vi "Table_BCK_Push.vi"(8 "error in (no error)":errorcluster, 11 "index":i32) -> (0 "Tables[]":string[](array[string]), 3 "Table Name":string)   [LabVIEW 2020]
uses:
  MS SQL/MS_Global.vi
panel:
  out "error out":errorcluster
  # "BCK_OP80_08_ASR"
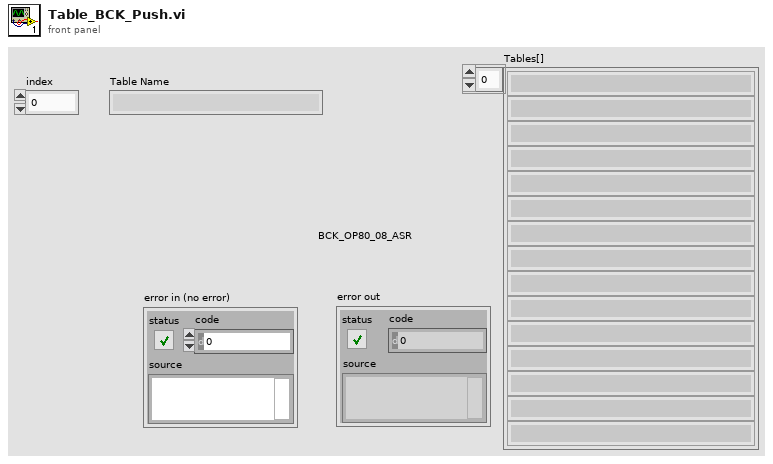
[diagram p1: front panel]
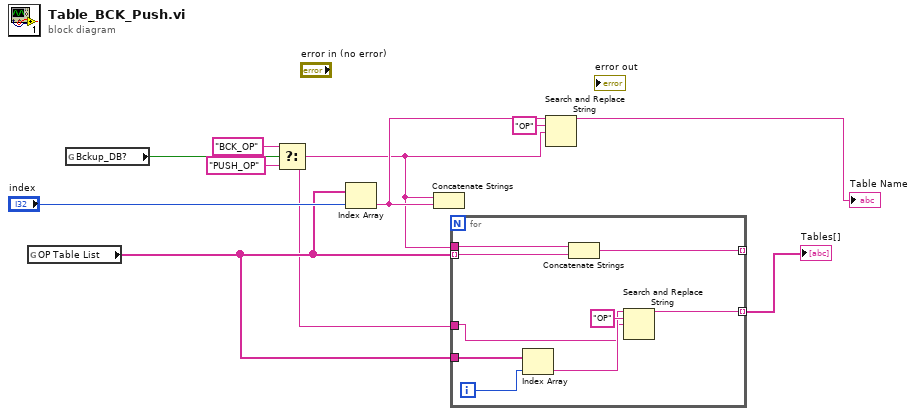
[diagram p0: block diagram]
diagram:
  n1 = global read "MS_Global.vi" "OP Table List"() -> (w5:string[])
  n2 = global read "MS_Global.vi" "Bckup_DB?"() -> (w7:bool)
  n3 = Select(t="BCK_OP", s=w7, f="PUSH_OP") -> (s? t:f=w2:string)
  n4 = Index Array(array=w5, index="index") -> (element=w3:string)
  n5 = Concatenate Strings(w2, w3) -> ()  [unwired: 1 out]
  n6 = for {
    tunnel: w5 -> [w15] mode=indexing
    tunnel: w2 -> [w19]
    tunnel: [w18] -> _ mode=indexing
    tunnel: w2 -> [w11]
    tunnel: [w16] -> w6 mode=indexing
    tunnel: w5 -> [w14]
    i -> [w13]
    n7 = Index Array(array=w14, index=w13) -> (element=w12:string)
    n8 = Concatenate Strings(w19, w15) -> (w18:string)
    n9 = Search and Replace String(input string=w12, search string="OP", replace string=w11) -> (result string=w16:string)  [unwired: 5 in, 3 out]
  }
  "Tables[]" <- w6
  n10 = Search and Replace String(input string=w3, search string="OP", replace string=w2) -> (result string=→"Table Name":string)  [unwired: 5 in, 3 out]
